vi "Post-Build Action.vi"(5 "Files Generated by Build":path[](array[path]), 6 "Top Level/Always Included VIs":path[](array[path]), 7 "Destination Path":path, 8 "error in (no error)":errorcluster, 9 "Target Name":string, 10 "Build Specification Name":string, 11 "Project Path":path) -> (0 "error out":errorcluster)   [LabVIEW 2021, in "Efficiency Sweep_Class D Amplifier.lvlib"]
uses:
  Efficiency Sweep_Class D Amplifier.lvlib
  MeasurementPlugin.lvclass
  <vilib>/MeasurementLink/MeasurementLink Measurement Server/MeasurementLink Measurement Server.lvlib
  C:/Program Files/National Instruments/LabVIEW 2021/vi.lib/MeasurementLink/MeasurementLink Measurement Server/Measurement Plugin Service/Measurement Plugin Service.lvclass
  C:/dev/class-d-amplifier/source/efficiency sweep/Efficiency Sweep_Class D Amplifier/Advanced/MeasurementPlugin.lvclass
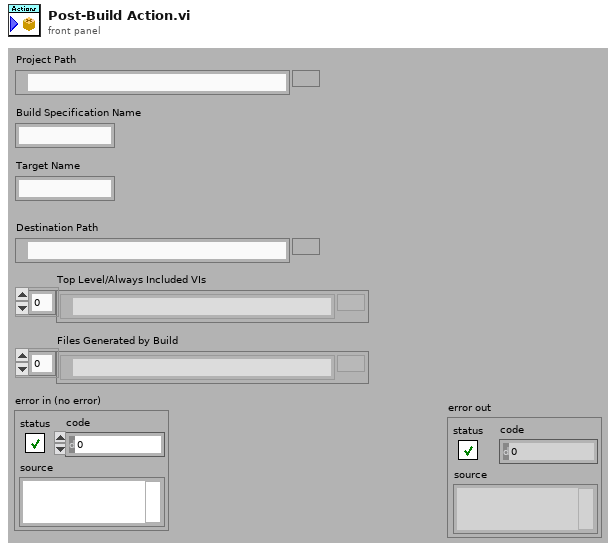
[diagram p1: front panel]
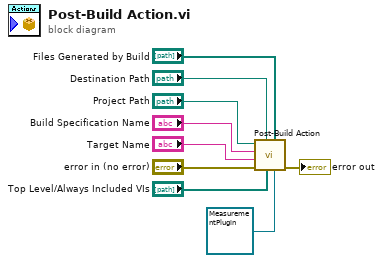
[diagram p0: block diagram]
diagram:
  n1 = call <vilib>:"Post-Build Action.vi"("measurement plugin service"=refnum<class "MeasurementPlugin.lvclass"> refnum ("MeasurementLink Measurement Template.lvlib:MeasurementPlugin.lvclass"), "files generated by build"="Files Generated by Build", "top level/always included VIs"="Top Level/Always Included VIs", "destination path"="Destination Path", "error in"="error in (no error)", "target name"="Target Name", "build specification name"="Build Specification Name", "project path"="Project Path") -> ("error out"=→"error out":errorcluster)  [unwired: 3 in]
